vi "Create Full Frequency Steps Array.vi"(9 "Fine region centers":dbl[](array[numeric]), 10 "Leading steps to wait":i32=5, 11 "Spectrum Recorder Configuration":T1={"Start frequency"=500000.0, "End frequency"=2000000.0, "Coarse step"=100.0, "Step duration"=0.004, "Red Pitaya address"="192.168.1.100", "Open plot \non start"=FALSE, "Regions width"=2000.0, "Fine step"=1.0, "Pause between scans"=0.0, "Clear rgs on start"=FALSE, "Output amplitude"=1.0, "Append measurements"=[], "Full scan period"=nan, "Full start"=500000.0, "Full end"=2000000.0, "Full step"=100.0} {"Full step" format="%#_6pHz"; "Full end" format="%#_6pHz"; "Full start" format="%#_6pHz"; "Full scan period" format="%#_6fm"; "Output amplitude" min=0.0 max=1.0 step=0.1 format="%#_6pV"; "Pause between scans" format="%#_6ps"; "Fine step" min=0.001 format="%#_6pHz"; "Regions width" format="%#_6pHz"; "Step duration" format="%#_6ps"; "Coarse step" format="%#_6pHz"; "End frequency" format="%#_6pHz"; "Start frequency" format="%#_6pHz"}) -> (3 "Steps":dbl[](array[numeric]) format="%#_8p")   [LabVIEW 2021]
uses:
  NHMFL_Core/Libraries/Red Pitaya/RP Core/Red Pitaya Transceiver Driver/Spectrum Configuration.ctl
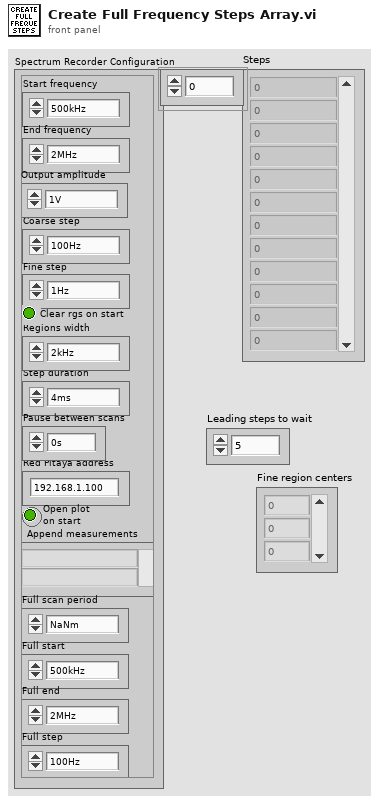
[diagram p1: front panel]
types:
  T1 = typedef "Spectrum Configuration.ctl" = cluster{"Start frequency":dbl, "End frequency":dbl, "Coarse step":dbl, "Step duration":dbl, "Red Pitaya address":string, "Open plot \non start":bool, "Regions width":dbl, "Fine step":dbl, "Pause between scans":dbl, "Clear rgs on start":bool, "Output amplitude":dbl, "Append measurements":string[], "Full scan period":dbl, "Full start":dbl, "Full end":dbl, "Full step":dbl}
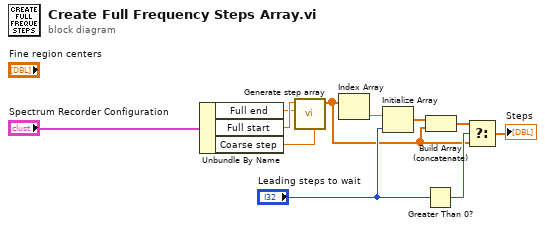
[diagram p0: block diagram]
diagram:
  n1 = Unbundle By Name("Spectrum Recorder Configuration") -> ("Full end"=w10:dbl, "Full start"=w11:dbl, "Coarse step"=w8:dbl)
  n2 = call "Generate step array.vi"("Step"=w8, "End"=w10, "Start"=w11) -> ("Steps"=w2:dbl[])  [unwired: 8 in]
  n3 = Index Array(array=w2) -> (element=w7:dbl)  [unwired: 1 in]
  n4 = Initialize Array(w7, "Leading steps to wait") -> (w4:dbl[])
  n5 = Greater Than 0?(x="Leading steps to wait") -> (x > 0?=w5:bool)
  n6 = Build Array (concatenate)(w4, w2) -> (w3:dbl[])
  n7 = Select(t=w3, s=w5, f=w2) -> (s? t:f=→"Steps":dbl[])
